vi "Challenge1SA.vi"() -> ()   [LabVIEW 2014, in "Challenge1SA.lvrbt"]
uses:
  Challenge1SA.lvrbt
  <vilib>/NXT/Block Support/NXT_InputPort.ctl
  <vilib>/NXT/Block Support/NXT_OutputPort.ctl
  <vilib>/NXT/Dual Mode Library/Sensors/EV3_Ultrasonic_IN.vi
  <vilib>/NXT/NXTIO Xnodes/NXTIONodeSubVIs/NXTMoveMotors.vi
  <vilib>/NXT/NXTIO Xnodes/NXTIONodeSubVIs/NXTStopMotors.vi
  <vilib>/NXT/Dual Mode Library/Waits/Wait_Num.vi
  <vilib>/NXT/Subs/LVHSConnector.ctl
  <vilib>/NXT/NXTIO Xnodes/AddressXNode/NXTIOAddress.xnode
  <vilib>/NXT/NXTIO Xnodes/NXTIOXNode/NXTIO.xnode
  <vilib>/NXT/LegoClasses/BrickReference/BrickReference.lvclass
panel:
  in  "stop":bool
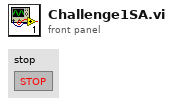
[diagram p1: front panel]
types:
  T1 = typedef "NXT_OutputPort.ctl" = u8
  T2 = typedef "NXT_InputPort.ctl" = u32
  T3 = typedef "LVHSConnector.ctl" = refnum<class "BrickReference.lvclass">
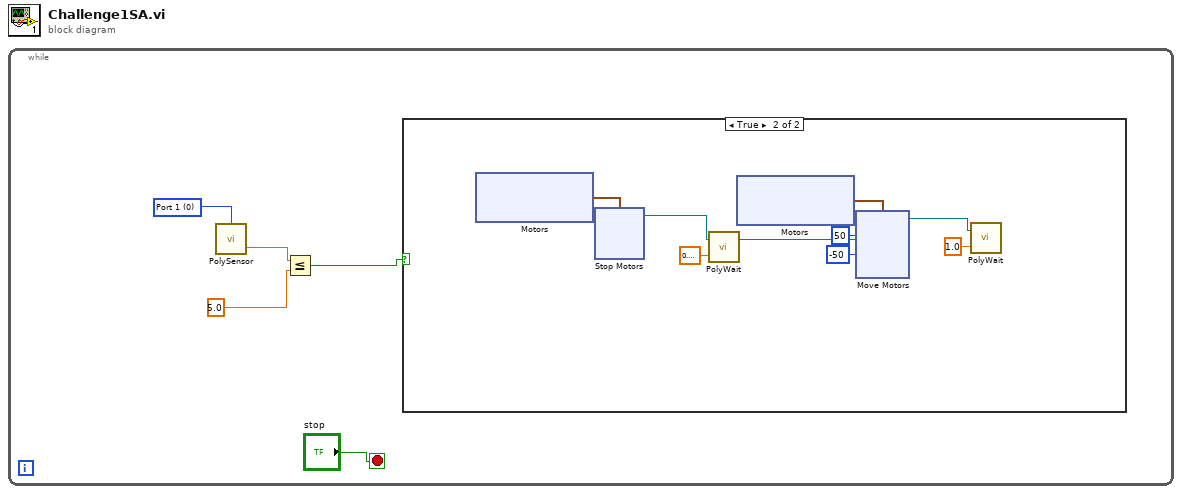
[diagram p0: block diagram]
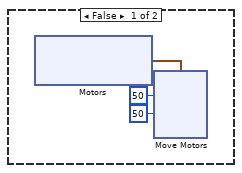
[diagram p2: hidden frame]
diagram:
  n1 = while {
    stop <- "stop" stop-if-true
    w4 = T2 0 items=["Port 1", "Port 2", "Port 3", "Port 4"] ("Port (Port 1)")
    n2 = call-poly <vilib>:"PolySensor.vi"("Port (Port 1)"=w4) -> ("Inches"=w3:sgl)  [unwired: 2 in, 1 out]
    n3 = Less Or Equal?(x=w3, y=sgl 5.0 ("Inches")) -> (x <= y?=w1:bool)
    n4 = case shown="True" w1 {
      frame False {
        n5 = xnode "Motors"() -> ("Motor"=w8:cluster{"Port":T1, "Port":T1})
        n6 = xnode "Move Motors"("Power/Speed 2"=i8 50, "Power/Speed 1"=i8 50, "Motors"=w8) -> ()  [unwired: 1 in, 1 out]
      }
      frame True {
        n7 = xnode "Motors"() -> ("Motor"=w26:cluster{"Port":T1, "Port":T1})
        n8 = xnode "Stop Motors"("Motors"=w26) -> ("NXT/EV3"=w23:T3)  [unwired: 1 in]
        n9 = call-poly <vilib>:"PolyWait.vi"("Time (1 sec)"=sgl 0.2, "NXT/EV3"=w23) -> ("NXT/EV3"=w22:T3)  [unwired: 2 in]
        n10 = xnode "Motors"() -> ("Motor"=w25:cluster{"Port":T1, "Port":T1})
        n11 = xnode "Move Motors"("Power/Speed 2"=i8 -50, "Power/Speed 1"=i8 50, "Motors"=w25, "NXT/EV3"=w22) -> ("NXT/EV3"=w19:T3)
        n12 = call-poly <vilib>:"PolyWait.vi"("Time (1 sec)"=sgl 1.0, "NXT/EV3"=w19) -> ()  [unwired: 2 in, 1 out]
      }
    }
  }
